vi "Close.vi"(8 "error in (no error)":errorcluster, 11 "NI DMM4072 in":refnum<class "NI DMM4072.lvclass">) -> (0 "error out":errorcluster, 3 "NI DMM4072 out":refnum<class "NI DMM4072.lvclass">)   [LabVIEW 2021, in "Concrete.lvlib" / "NI DMM4072.lvclass"]
uses:
  NI DMM4072.lvclass
  NI DMM4072.lvclass/NI DMM4072.ctl
  Harware Abstraction/MultiIO/MultiFunction IO.lvclass
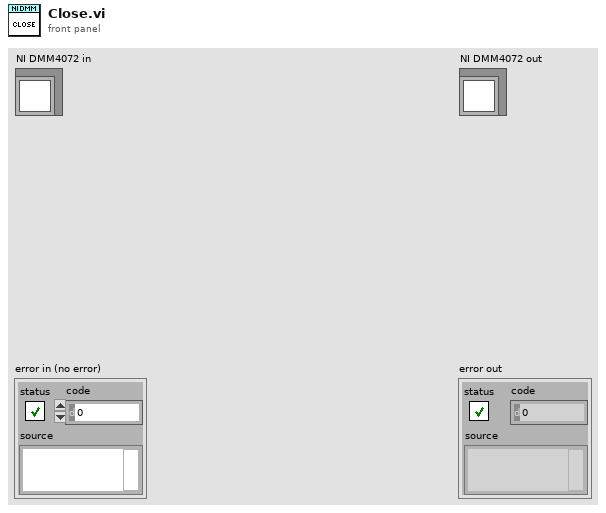
[diagram p1: front panel]
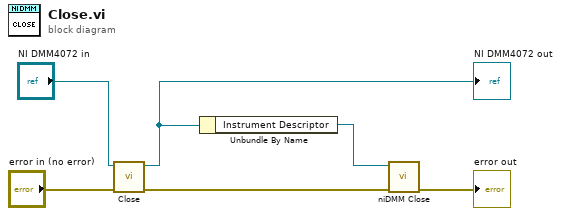
[diagram p0: block diagram]
diagram:
  n1 = call-parent "Close.vi"("error in (no error)"="error in (no error)", "Instrument in"="NI DMM4072 in") -> ("error out"=w4:errorcluster, "Instrument out"=w2:refnum<class "NI DMM4072.lvclass">)  [unwired: 8 in]
  "NI DMM4072 out" <- w2
  n2 = Unbundle By Name(w2) -> ("Instrument Descriptor"=w1:refnum<k15>)
  n3 = call <instrlib>:"niDMM Close.vi"("error in (no error)"=w4, "instrument handle"=w1) -> ("error out"=→"error out":errorcluster)  [unwired: 9 in]
